vi "Destroy All Message Queues.vi"(8 "error in (no error)":errorcluster, 11 "Message Queues Out":T1) -> (0 "error out":errorcluster)   [LabVIEW 2014, in "WINFAS 2 Message Queue.lvlib"]
doc: "This VI creates and initializes all the message queues for your application. If your application requires more than one message queue, right-click the \"Message Queues\" constant above and select Open Type Def. Add the new Message Queue(s) to the type definition, then initialize them in this VI."
uses:
  WINFAS 2 Message Queue.lvlib
  All Message Queues.ctl
  Message Cluster.ctl
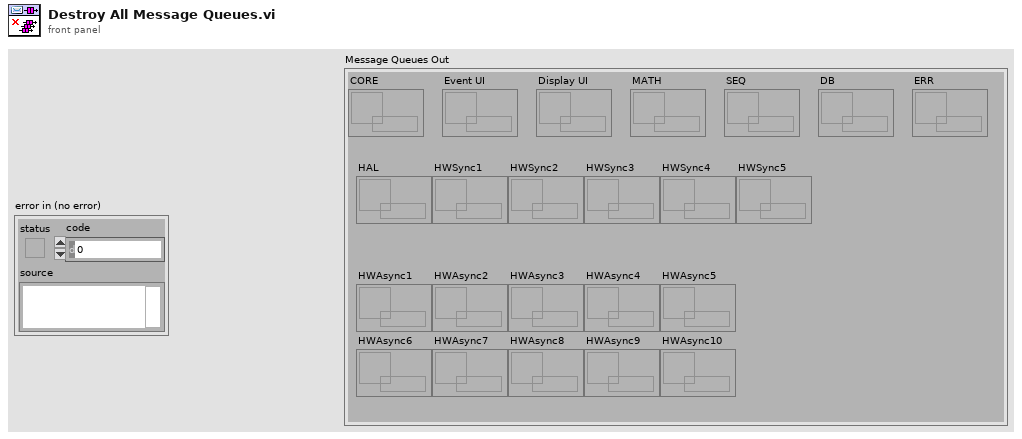
[diagram p1: front panel]
types:
  T1 = typedef "WINFAS 2 Message Queue.lvlib/All Message Queues.ctl" = cluster{"CORE":refnum<queue>, "Event UI":refnum<queue>, "Display UI":refnum<queue>, "MATH":refnum<queue>, "SEQ":refnum<queue>, "DB":refnum<queue>, "ERR":refnum<queue>, "HAL":refnum<queue>, "HWSync1":refnum<queue>, "HWSync2":refnum<queue>, "HWSync3":refnum<queue>, "HWSync4":refnum<queue>, "HWSync5":refnum<queue>, "HWAsync1":refnum<queue>, "HWAsync2":refnum<queue>, "HWAsync3":refnum<queue>, "HWAsync4":refnum<queue>, "HWAsync5":refnum<queue>, "HWAsync6":refnum<queue>, "HWAsync7":refnum<queue>, "HWAsync8":refnum<queue>, "HWAsync9":refnum<queue>, "HWAsync10":refnum<queue>}
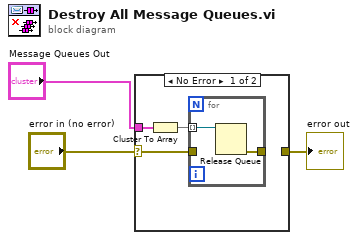
[diagram p0: block diagram]
diagram:
  n1 = case shown="No Error" "error in (no error)" {
    selector: "error in (no error)" -> [w4 w9]
    tunnel: [_ w9] -> w3
    tunnel: "Message Queues Out" -> [w6 _]
    frame No Error {
      n2 = Cluster To Array(cluster=w6) -> (array=w5:refnum<queue>[])
      n3 = for {
        tunnel: w5 -> [w8] mode=indexing
        tunnel: w4 -> [_]
        tunnel: [w7] -> _
        n4 = Release Queue(queue=w8) -> (error out=w7:errorcluster)  [unwired: 2 in, 2 out]
      }
    }
    frame Error {
    }
  }
  "error out" <- w3
